vi "Flash_replace.vi"(8 "error in":errorcluster, 10 "Array":string[](array[string])=["COM50", "D:\\Users\\A. Halstesd Evander\\Documents\\DTU_Manual_Flash\\Info\\Configuration\\RX01_DTU_N58_Application_0_0_10.pac", "E:\\Users\\A. Halstesd Evander\\Downloads\\RESEARCHDOWNLOAD_R22.19.1701\\RESEARCHDOWNLOAD_R22.19.1701\\Bin\\CmdDloader.exe", "F:\\Users\\A. Halstesd Evander\\Downloads\\RESEARCHDOWNLOAD_R22.19.1701\\RESEARCHDOWNLOAD_R22.19.1701\\Bin\\result.txt"], 11 "file path (use dialog)":path) -> (0 "error out":errorcluster)   [LabVIEW 2024, in "SSL_Certification.lvlib"]
uses:
  SSL_Certification.lvlib
panel:
  out "String":string
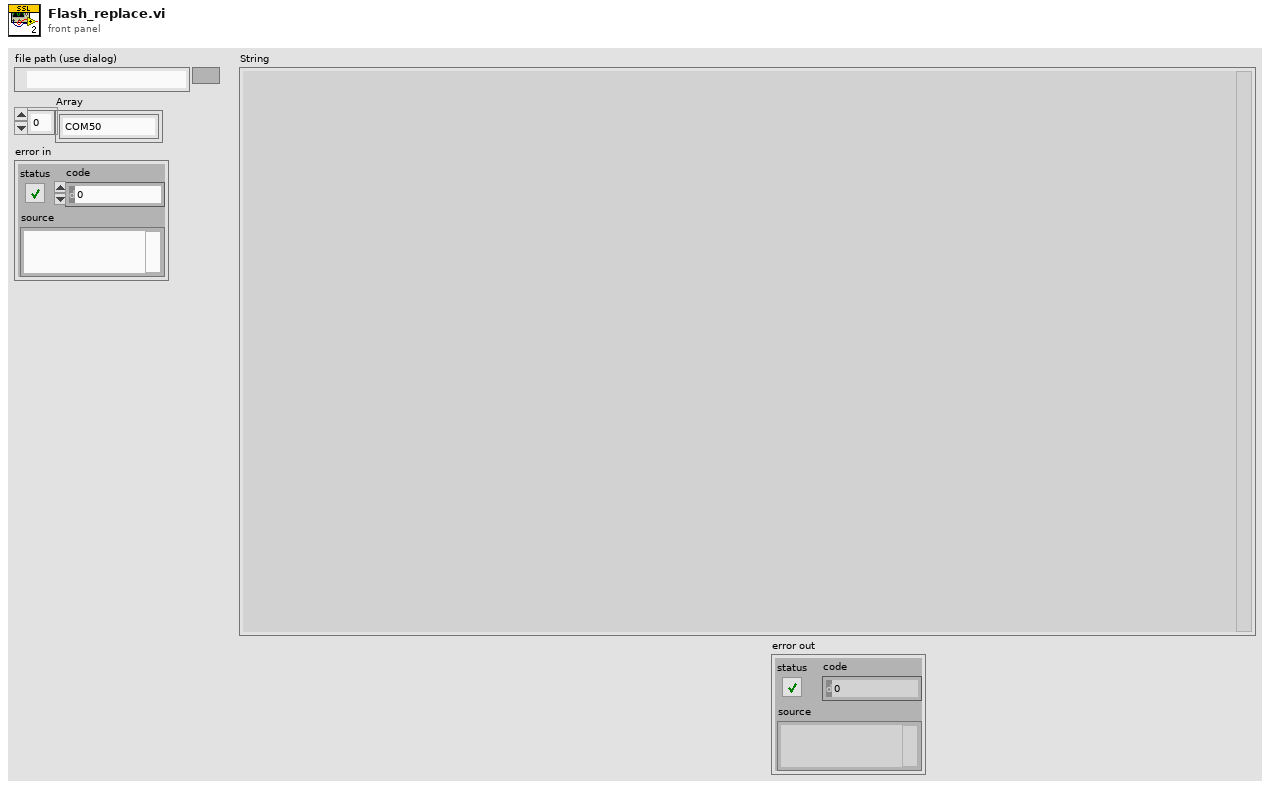
[diagram p1: front panel]
types:
  T1 = enum16{"open", "replace", "create", "open or create", "replace or create", "replace or create with confirmation"}
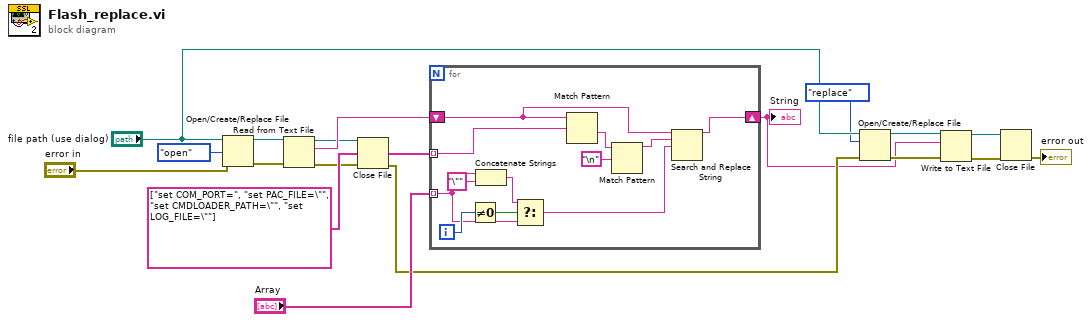
[diagram p0: block diagram]
diagram:
  n1 = Open/Create/Replace File(file path (use dialog)="file path (use dialog)", error in="error in", operation (0:open)=T1."open") -> (refnum out=w16:refnum<file>, error out=w17:errorcluster)  [unwired: 3 in, 1 out]
  n2 = Read from Text File(file (use dialog)=w16, error in=w17) -> (refnum out=w11:refnum<file>, text=w14:string, error out=w12:errorcluster)  [unwired: 2 in, 1 out]
  n3 = Close File(refnum=w11, error in=w12) -> (error out=w8:errorcluster)  [unwired: 1 out]
  n4 = for {
    tunnel: string[] ["set COM_PORT=", "set PAC_FILE=\"", "set CMDLOADER_PATH=\"", "set LOG_FILE=\""] -> [w30] mode=indexing
    shift-right: [w22] -> w3
    shift-left: w14 -> [w29]
    tunnel: "Array" -> [w25] mode=indexing
    i -> [w27]
    n5 = Not Equal To 0?(x=w27) -> (x != 0?=w28:bool)
    n6 = Concatenate Strings(w25, "\"" ("string")) -> (w26:string)
    n7 = Select(t=w26, s=w28, f=w25) -> (s? t:f=w23:string)
    n8 = Match Pattern(string=w29, regular expression=w30) -> (after substring=w21:string)  [unwired: 1 in, 3 out]
    n9 = Match Pattern(string=w21, regular expression="\n") -> (before substring=w19:string)  [unwired: 1 in, 3 out]
    n10 = Search and Replace String(input string=w29, search string=w19, replace string=w23) -> (result string=w22:string)  [unwired: 5 in, 3 out]
  }
  "String" <- w3
  n11 = Open/Create/Replace File(file path (use dialog)="file path (use dialog)", error in=w8, operation (0:open)=T1."replace") -> (refnum out=w7:refnum<file>, error out=w6:errorcluster)  [unwired: 3 in, 1 out]
  n12 = Write to Text File(file (use dialog)=w7, text=w3, error in=w6) -> (refnum out=w4:refnum<file>, error out=w5:errorcluster)  [unwired: 1 in, 1 out]
  n13 = Close File(refnum=w4, error in=w5) -> (error out=→"error out":errorcluster)  [unwired: 1 out]
